vi "Trigger.vi"(8 "error in (no error)":errorcluster, 11 "Instrument Actor in":refnum<class "Instrument Actor.lvclass">) -> (0 "error out":errorcluster, 3 "Instrument Actor out":refnum<class "Instrument Actor.lvclass">)   [LabVIEW 2016, in "Instrument Actor.lvclass"]
uses:
  Instrument Actor.lvclass
  C:/github/LabActor/Worker/Worker.lvclass
  Worker/Worker.lvclass/Worker.ctl
  Instrument Actor.lvclass/Instrument Actor.ctl
  Read Instrument driver.vi
  Write Instrument driver.vi
  Template Module/Read State.vi
  NHMFL_Core/Libraries/Instruments/Instrument Driver/Instrument Driver.lvclass
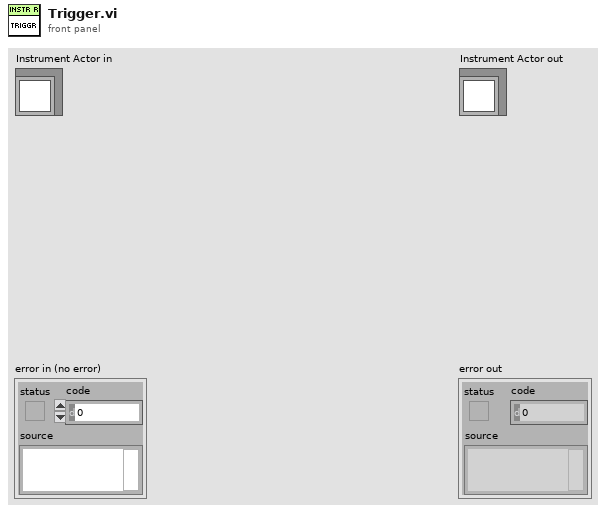
[diagram p1: front panel]
types:
  T1 = typedef "Worker State.ctl" = enum16{"Idle", "Starting", "Working", "Stopping"}
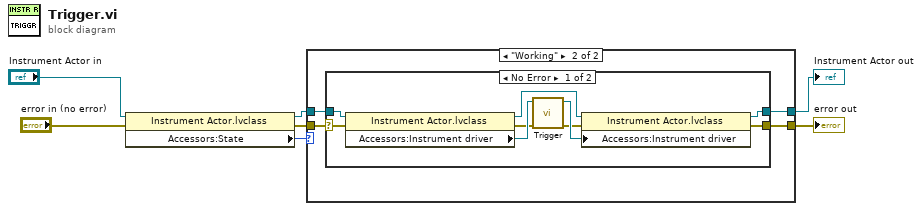
[diagram p0: block diagram]
diagram:
  n1 = property class="Instrument Actor.lvclass"(reference="Instrument Actor in", error in="error in (no error)") -> (reference out=w5:refnum<class "Instrument Actor.lvclass">, error out=w6:errorcluster, "Accessors:State"=w7:T1)
  n2 = case shown="\"Working\"" w7 {
    tunnel: [w8 w13] -> w2
    tunnel: [w9 w12] -> w1
    tunnel: w5 -> [w9 w11]
    tunnel: w6 -> [w8 w10]
    frame "Idle", Default {
    }
    frame "Working" {
      n3 = case shown="No Error" w10 {
        selector: w10 -> [w14 w24]
        tunnel: [w17 w24] -> w13
        tunnel: [w16 w23] -> w12
        tunnel: w11 -> [w15 w23]
        frame No Error {
          n4 = property class="Instrument Actor.lvclass"(reference=w15, error in=w14) -> (reference out=w20:refnum<class "Instrument Actor.lvclass">, error out=w21:errorcluster, "Accessors:Instrument driver"=w22:refnum<class "Instrument Driver.lvclass">)
          n5 = call-dynamic "Trigger.vi"("error in (no error)"=w21, "Instrument Driver in"=w22) -> ("error out"=w18:errorcluster, "Instrument Driver out"=w19:refnum<class "Instrument Driver.lvclass">)  [unwired: 8 in]
          n6 = property class="Instrument Actor.lvclass"(reference=w20, error in=w18, "Accessors:Instrument driver"=w19) -> (reference out=w16:refnum<class "Instrument Actor.lvclass">, error out=w17:errorcluster)
        }
        frame Error {
        }
      }
    }
  }
  "error out" <- w2
  "Instrument Actor out" <- w1
